vi "Select state.vi"(2 "Z3(State)":T1(array[ring])=[enum."stop ready", enum."stop ready", enum."stop ready", enum."stop ready"], 3 "Order":u32[](array[numeric])=[1, 2, 3, 4], 4 "N_pump_on_ref":u32=1, 5 "Z2(StationSetState)":T2(ring)=enum."on") -> (0 "N_curr":i32, 1 "Z4(AutoSetState)":T1(array[ring]))   [LabVIEW 2019, in "Userlib.lvlib"]
uses:
  Userlib.lvlib
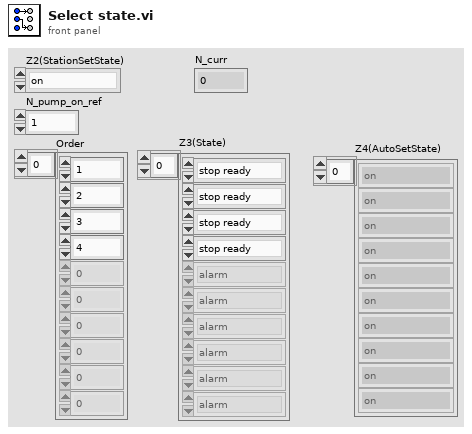
[diagram p1: front panel]
types:
  T1 = enum8{"alarm", "disabled", "not ready", "stop ready", "reserv", "switched off", "switched on", "check", "on min", "decrease speed", "on", "increase speed", "on max"}[]
  T2 = enum8{"alarm", "disabled", "not ready", "stop ready", "reserv", "switched off", "switched on", "check", "on min", "decrease speed", "on", "increase speed", "on max"}
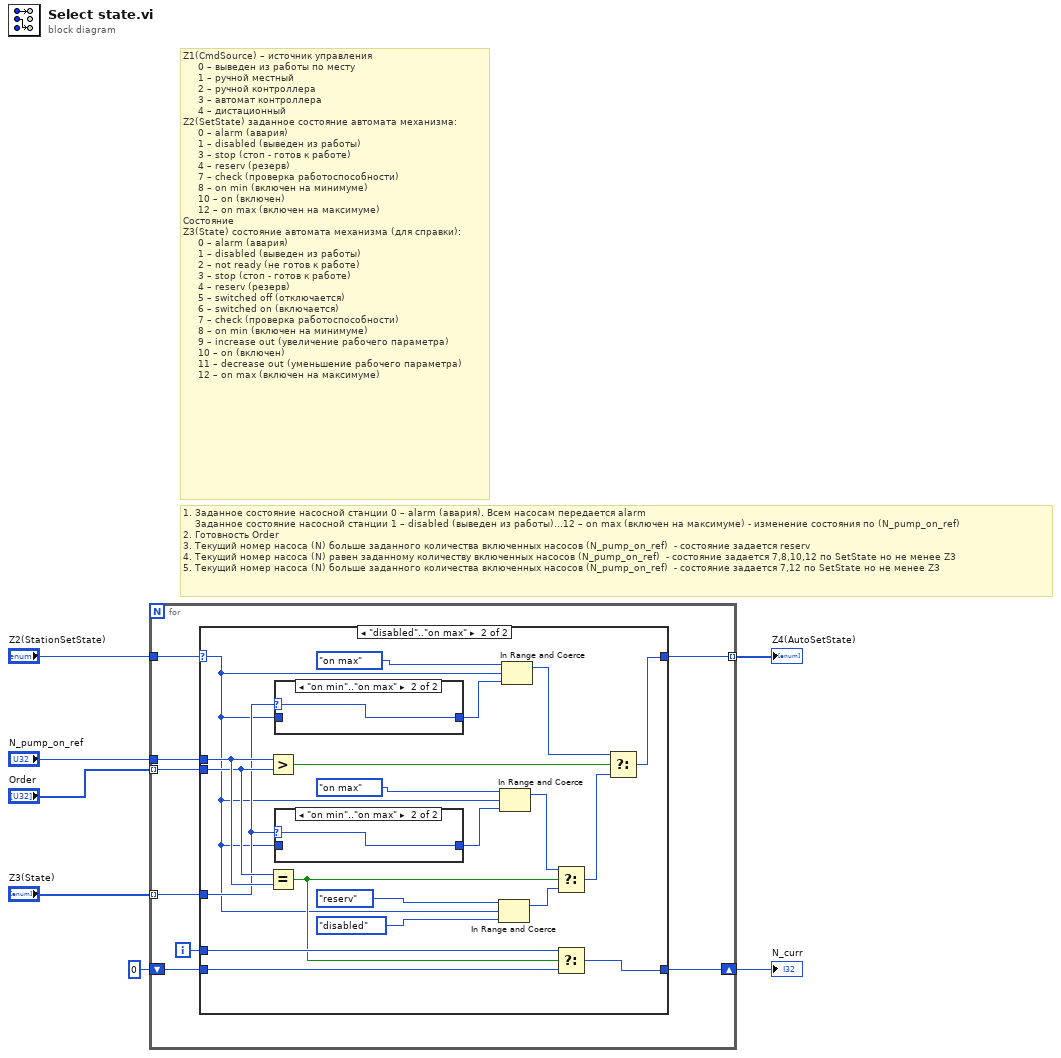
[diagram p0: block diagram]
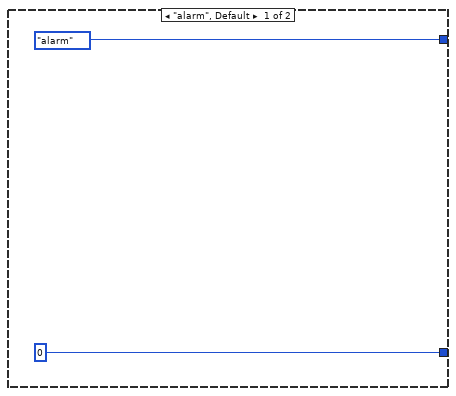
[diagram p2: hidden frame]
diagram:
  # "1. Заданное состояние насосной станции 0 – alarm (авария). Всем насосам передается alarm\n    Заданное состояние насосной станции 1 – disabled (выведен из работы)...12 – on max (включен на максимуме) - изменение состояния по (N_pump_on_ref)\n2. Готовность Order\n3. Текущий номер насоса (N) больше заданного количества включенных насосов (N_pump_on_ref)  - состояние задается reserv\n4. Текущий номер насоса (N) равен заданному количеству включенных насосов (N_pump_on_ref)  - состояние задается 7,8,10,12 по SetState но не менее Z3\n5. Текущий номер насоса (N) больше заданного количества включенных насосов (N_pump_on_ref)  - состояние задается 7,12 по SetState но не менее Z3"
  # "Z1(CmdSource) – источник управления\n     0 – выведен из работы по месту\n     1 – ручной местный\n     2 – ручной контроллера\n     3 – автомат контроллера\n     4 – дистационный\nZ2(SetState) заданное состояние автомата механизма:\n     0 – alarm (авария)\n     1 – disabled (выведен из работы)\n     3 – stop (стоп - готов к работе)\n     4 – reserv (резерв)\n     7 – check (проверка работоспособности)\n     8 – on min (включен на минимуме)\n     10 – on (включен)\n     12 – on max (включен на максимуме)\nСостояние\nZ3(State) состояние автомата механизма (для справки):\n     0 – alarm (авария)\n     1 – disabled (выведен из работы)\n     2 – not ready (не готов к работе)\n     3 – stop (стоп - готов к работе)\n     4 – reserv (резерв)\n     5 – switched off (отключается)\n     6 – switched on (включается)\n     7 – check (проверка работоспособности)\n     8 – on min (включен на минимуме)\n     9 – increase out (увеличение рабочего параметра)\n     10 – on (включен)\n     11 – decrease out (уменьшение рабочего параметра)\n     12 – on max (включен на максимуме)"
  n1 = for {
    tunnel: "N_pump_on_ref" -> [w15]
    tunnel: "Z2(StationSetState)" -> [w14]
    tunnel: "Order" -> [w13] mode=indexing
    tunnel: [w12] -> w4 mode=indexing
    shift-right: [w10] -> w2
    shift-left: 0 -> [w9]
    tunnel: "Z3(State)" -> [w8] mode=indexing
    i -> [w11]
    n2 = case shown="\"disabled\"..\"on max\"" w14 {
      selector: w14 -> [_ w19]
      tunnel: [T2."alarm" ("Z2(SetState) 2") w29] -> w12
      tunnel: w15 -> [_ w27]
      tunnel: w13 -> [_ w26]
      tunnel: w11 -> [_ w23]
      tunnel: [0 w25] -> w10
      tunnel: w9 -> [_ w24]
      tunnel: w8 -> [_ w20]
      frame "alarm", Default {
      }
      frame "disabled".."on max" {
        n3 = Greater?(x=w27, y=w26) -> (0:w30:bool)
        n4 = Equal?(x=w26, y=w27) -> (x = y?=w21:bool)
        n5 = case shown="\"on min\"..\"on max\"" w20 {
          selector: w20 -> [_ w41]
          tunnel: w19 -> [w40 _]
          tunnel: [w40 w41] -> w22
          frame "alarm".."reserv", Default {
          }
          frame "on min".."on max" {
          }
        }
        n6 = case shown="\"on min\"..\"on max\"" w20 {
          selector: w20 -> [_ w39]
          tunnel: w19 -> [w38 _]
          tunnel: [w38 w39] -> w18
          frame "alarm".."reserv", Default {
          }
          frame "on min".."on max" {
          }
        }
        n7 = In Range and Coerce(upper limit=T2."reserv" ("Z2(SetState) 2"), x=w19, lower limit=T2."disabled" ("Z2(SetState) 2")) -> (coerced(x)=w28:T2)  [unwired: 1 out]
        n8 = In Range and Coerce(upper limit=T2."on max" ("Z2(SetState) 2"), x=w19, lower limit=w18) -> (coerced(x)=w34:T2)  [unwired: 1 out]
        n9 = In Range and Coerce(upper limit=T2."on max" ("Z2(SetState) 2"), x=w19, lower limit=w22) -> (coerced(x)=w32:T2)  [unwired: 1 out]
        n10 = Select(t=w34, s=w21, f=w28) -> (s? t:f=w31:T2)
        n11 = Select(t=w23, s=w21, f=w24) -> (s? t:f=w25:i32)
        n12 = Select(t=w32, s=w30, f=w31) -> (s? t:f=w29:T2)
      }
    }
  }
  "Z4(AutoSetState)" <- w4
  "N_curr" <- w2
